vi "EditorDaemon editScript.vi"(8 "error in (no error)":errorcluster) -> (0 "error out":errorcluster)   [LabVIEW 2018]
uses:
  PC/winForms/winForms editorType.ctl
  ctl/editScriptState.ctl
  C:/ATI_MS_InstrumentControl/dll/ScintillaNET.dll
  dll/ScintillaNET.dll
  PC/PublicSubVI/Class/QMH/QMH.lvclass
  System.Windows.Forms
panel:
  in  "saveAsBtn":bool
  in  "openBtn":bool
  in  "searchStr":string caption="Search :"
  in  "script":refnum<k24>(container)
  in  "msgListbox":i32(listbox)
  in  "stop":bool
  in  "cancelBtn":bool
  in  "submitBtn":bool
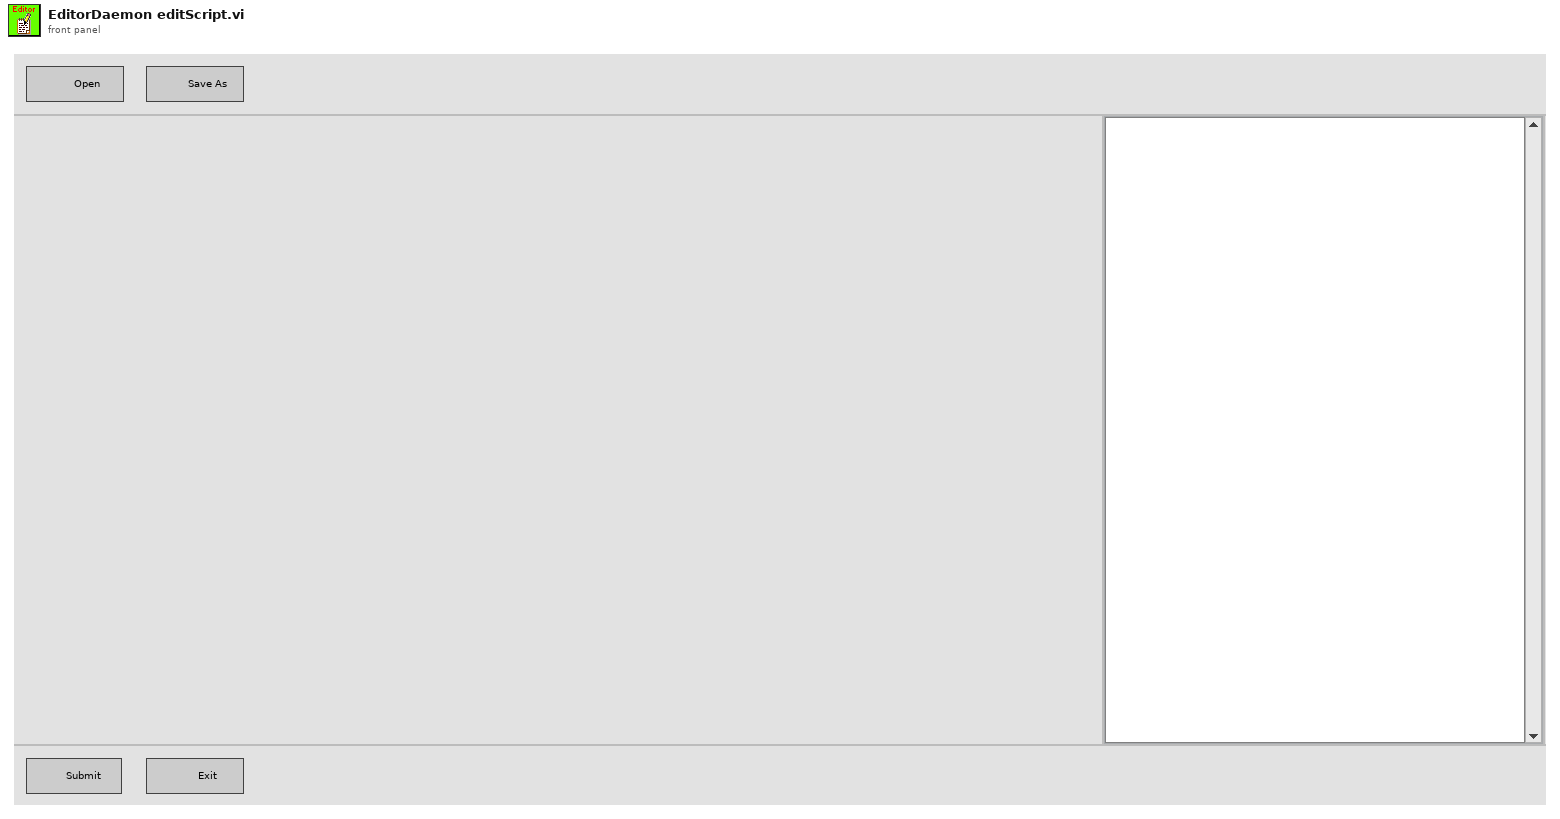
[diagram p1: front panel]
types:
  T1 = typedef "editScriptState.ctl" = enum16{"init", "loadScript", "newScript", "runScript", "close"}
  T2 = typedef "winForms editorType.ctl" = enum16{"Recipe", "SigProc", "Editor"}
  T3 = typedef "eventvkey.ctl" = enum16{"ASCII", "Enter", "Return", "Shift", "Ctrl", "Alt", "Cmd", "Opt", "Caps", "NumLock", "Clear", "Break", "Up", "Down", "Left", "Right", "Insert", "Delete", "Home", "End", "PageUp", "PageDown", "Escape", "Help", "Pause", "ScrollLock", "F1", "F2", "F3", "F4", "F5", "F6", "F7", "F8", "F9", "F10", "F11", "F12", "F13", "F14", "F15", "F16", "F17", "F18", "F19", "F20", "F21", "F22", "F23", "F24", "Play", "VolumeUp", "VolumeDown", "Mute", "Two Byte Char"}
  T4 = enum16{"open", "replace", "create", "open or create", "replace or create", "replace or create with confirmation"}
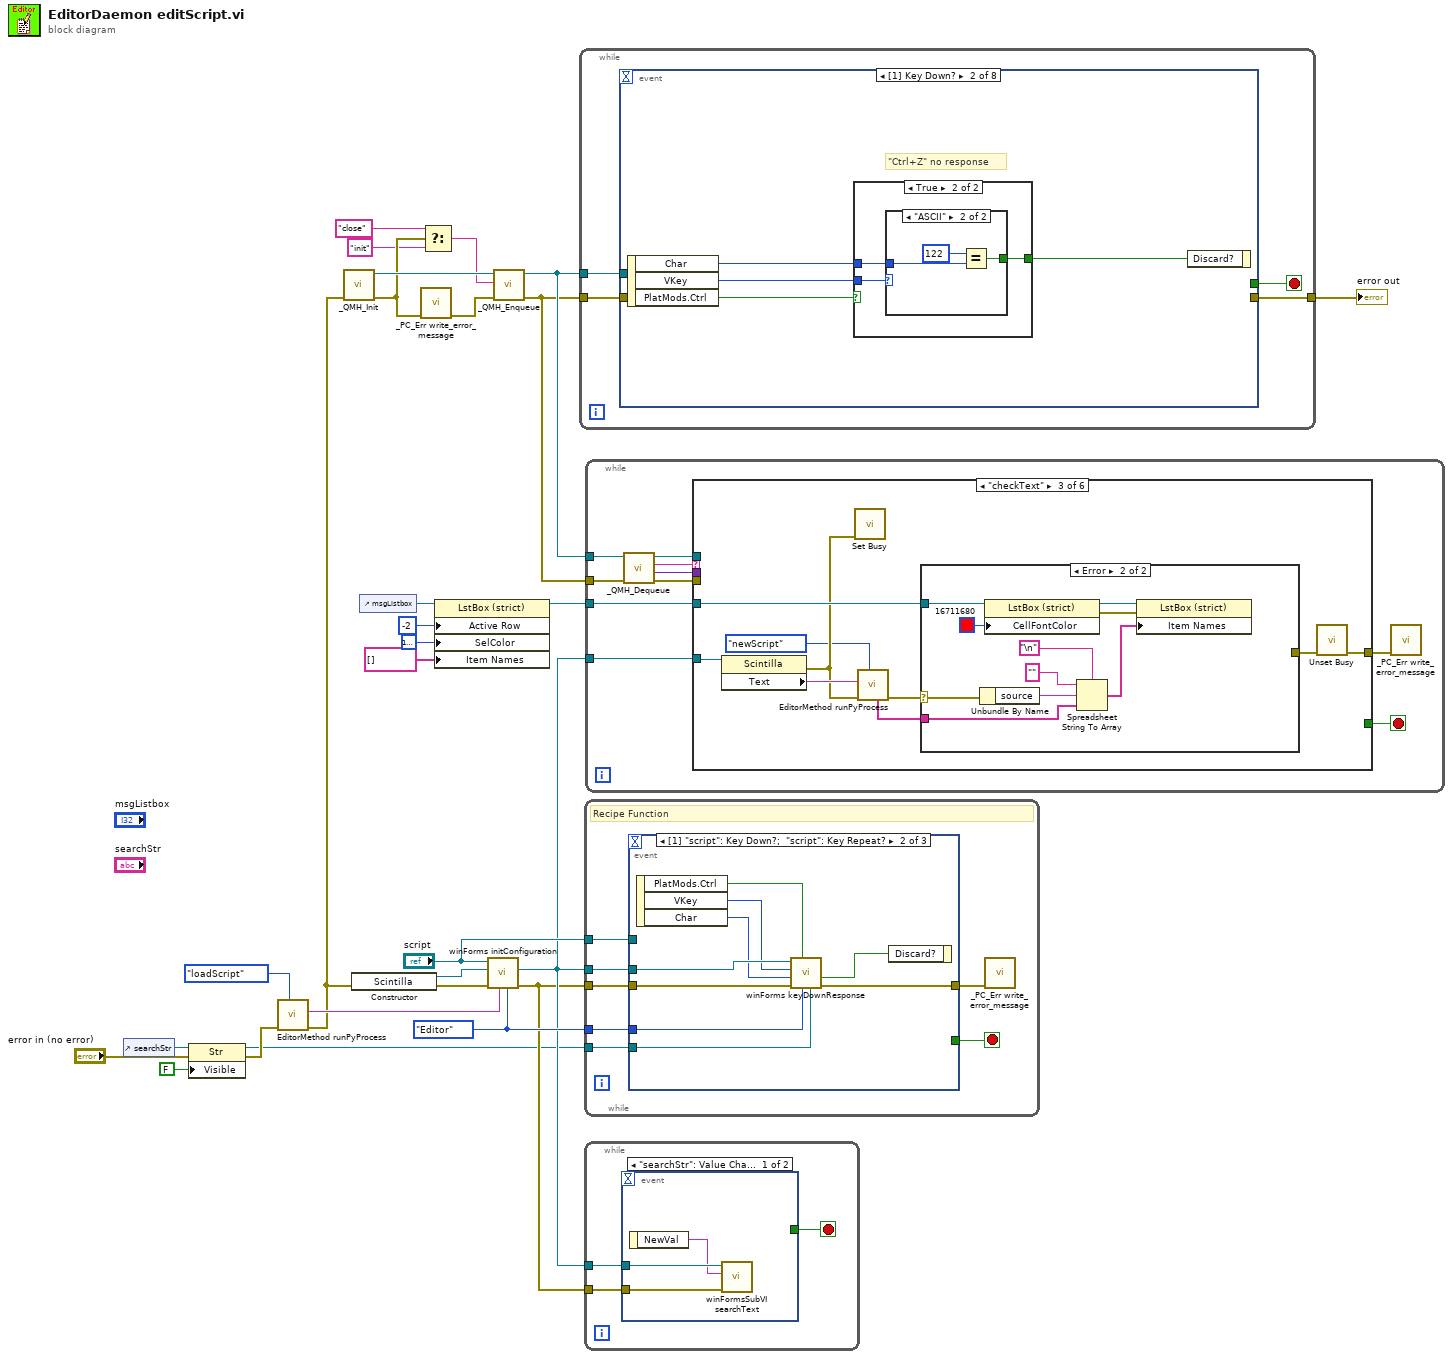
[diagram p0: block diagram]
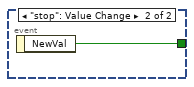
[diagram p2: hidden frame]
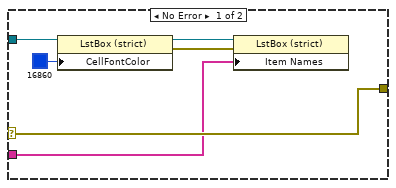
[diagram p5: hidden frame]
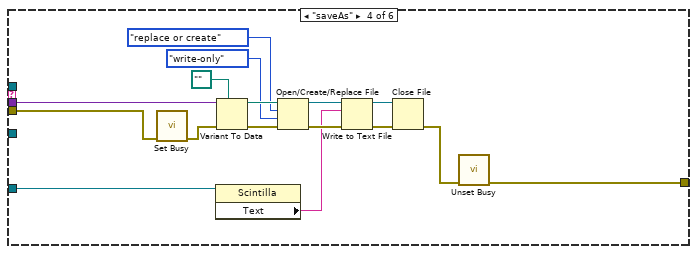
[diagram p6: hidden frame]
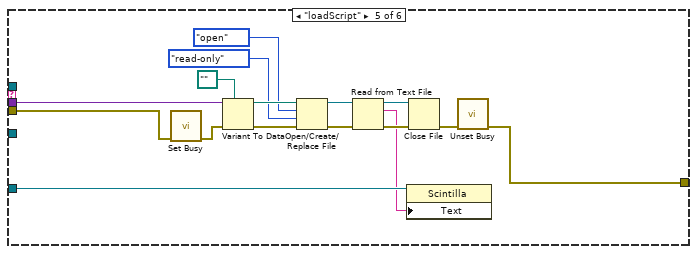
[diagram p7: hidden frame]
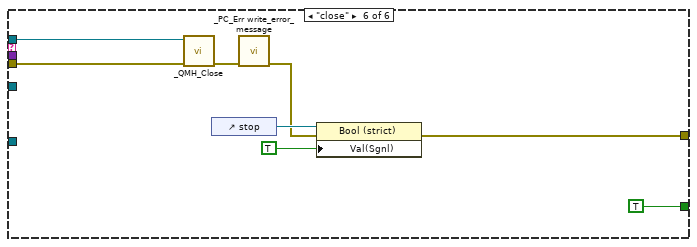
[diagram p8: hidden frame]
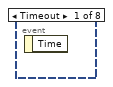
[diagram p9: hidden frame]
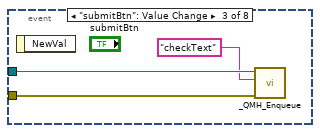
[diagram p12: hidden frame]
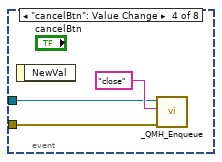
[diagram p13: hidden frame]
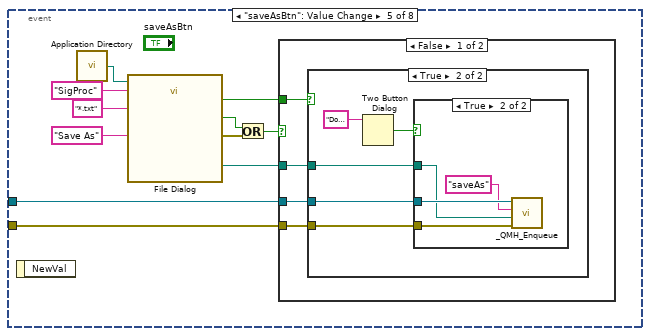
[diagram p14: hidden frame]
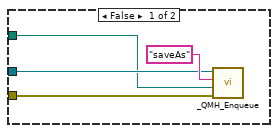
[diagram p15: hidden frame]
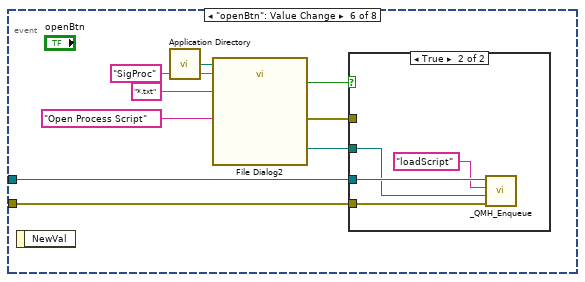
[diagram p18: hidden frame]
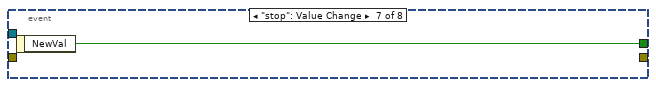
[diagram p20: hidden frame]
diagram:
  w19 = winForms_editorType."Editor" ("editorType")
  n1 = control-ref of="searchStr"() -> (w9:refnum<vi>)
  n2 = property class="Str"(reference=w9, error in="error in (no error)", "Visible"=FALSE) -> (reference out=w8:refnum<vi>, error out=w10:errorcluster)
  n3 = call "EditorMethod runPyProcess.vi"("func"=editScriptState."loadScript", "error in (no error)"=w10) -> ("error out"=w7:errorcluster, "pyCode"=w16:string)  [unwired: 6 in, 2 out]
  n4 = call "_QMH_Init.vi"("error in (no error)"=w7) -> ("error out"=w24:errorcluster, "QMH out"=w25:refnum<class "QMH.lvclass">)  [unwired: 9 in]
  n5 = constructor class="Scintilla"(error in=w7) -> (reference out=w28:refnum<k24>, error out=w27:errorcluster)  [unwired: 2 in, 1 out]
  n6 = control-ref of="msgListbox"() -> (w5:refnum<vi>)
  n7 = call "_PC_Err write_error_message.vi"("error in"=w24) -> ("error out"=w23:errorcluster)  [unwired: 10 in]
  n8 = Select(t="close", s=w24, f="init") -> (s? t:f=w22:string)
  n9 = property class="LstBox (strict)"(reference=w5, "Active Row"=-2 ("Active Row:Active Row Number"), "SelColor"=u32 16777226, "Item Names"=string[] []) -> (reference out=w4:refnum<vi>)  [unwired: 1 in, 1 out]
  n10 = call "winForms initConfiguration.vi"("editorType"=w19, "initText"=w16, "error in (no error)"=w27, "scintillaRefNum in"=w28, "panelRefNum"="script") -> ("error out"=w13:errorcluster, "scintillaRefNum out"=w14:refnum<k24>)  [unwired: 5 in]
  n11 = call "_QMH_Enqueue.vi"("error in (no error)"=w23, "Msg"=w22, "QMH in"=w25) -> ("error out"=w20:errorcluster, "QMH out"=w21:refnum<class "QMH.lvclass">)  [unwired: 7 in]
  n12 = while {
    tunnel: w21 -> [w31]
    tunnel: w20 -> [w30]
    tunnel: [w29] -> w15
    stop <- w32 stop-if-true
    n13 = event shown="[1] Key Down?" {
      selector: _ -> [_ _ _ _ _ _ _ _]
      dyn-events: _ -> [_ _ _ _ _ _ _ _]
      timeout: _ -> [_ _ _ _ _ _ _ _]
      tunnel: [_ _ _ _ _ _ w90 _] -> w32
      tunnel: w31 -> [_ _ w45 w47 w50 w78 _ w94]
      tunnel: w30 -> [_ _ w44 w46 w49 w77 _ w93]
      tunnel: [_ _ _ _ _ _ _ w91] -> w29
      event Timeout {
        n14 = event-data() -> ()  [unwired: 1 in, 1 out]
      }
      event Key Down? {
        # "\"Ctrl+Z\" no response"
        n15 = event-data() -> ("Char"=w34:i16, "VKey"=w35:T3, "PlatMods.Ctrl"=w36:bool)  [unwired: 1 in]
        n16 = case shown="True" w36 {
          tunnel: w35 -> [_ w39]
          tunnel: w34 -> [_ w38]
          tunnel: [_ w37] -> w33
          frame False {
          }
          frame True {
            n17 = case shown="\"ASCII\"" w39 {
              tunnel: w38 -> [_ w42]
              tunnel: [_ w40] -> w37
              frame "Escape", Default {
              }
              frame "ASCII" {
                n18 = Equal?(x=i16 122, y=w42) -> (x = y?=w40:bool)
              }
            }
          }
        }
        n19 = event-data("Discard?"=w33) -> ()  [unwired: 1 in, 1 out]
      }
      event "submitBtn": Value Change {
        n20 = event-data() -> ()  [unwired: 1 in, 1 out]
        n21 = call "_QMH_Enqueue.vi"("error in (no error)"=w44, "Msg"="checkText", "QMH in"=w45) -> ()  [unwired: 7 in, 2 out]
      }
      event "cancelBtn": Value Change {
        n22 = event-data() -> ()  [unwired: 1 in, 1 out]
        n23 = call "_QMH_Enqueue.vi"("error in (no error)"=w46, "Msg"="close", "QMH in"=w47) -> ()  [unwired: 7 in, 2 out]
      }
      event "saveAsBtn": Value Change {
        n24 = event-data() -> ()  [unwired: 1 in, 1 out]
        n25 = call <vilib>:"Application Directory.vi"() -> ("Application Directory"=w59:path)
        n26 = call "File Dialog"("start path"=w59, "prompt"="Save As", "default name"="SigProc" ("pattern label"), "pattern (all files)"="*.txt") -> ("selected path"=w54:path, "exists"=w55:bool, "cancelled"=w53:bool, "error out"=w52:errorcluster)  [unwired: 8 in]
        n27 = Or(x=w53, y=w52) -> (x .or. y?=w51:bool)
        n28 = case shown="False" w51 {
          tunnel: w55 -> [w63 _]
          tunnel: w54 -> [w62 _]
          tunnel: w50 -> [w61 _]
          tunnel: w49 -> [w60 _]
          frame False {
            n29 = case shown="True" w63 {
              tunnel: w62 -> [w64 w68]
              tunnel: w61 -> [w66 w70]
              tunnel: w60 -> [w65 w69]
              frame False {
                n30 = call "_QMH_Enqueue.vi"("error in (no error)"=w65, "Data"=w64, "Msg"="saveAs", "QMH in"=w66) -> ()  [unwired: 6 in, 2 out]
              }
              frame True {
                n31 = Two Button Dialog(message="Do you want to overwrite this file?") -> (T button?=w71:bool)  [unwired: 2 in]
                n32 = case shown="True" w71 {
                  tunnel: w70 -> [_ w76]
                  tunnel: w69 -> [_ w73]
                  tunnel: w68 -> [_ w75]
                  frame False {
                  }
                  frame True {
                    n33 = call "_QMH_Enqueue.vi"("error in (no error)"=w73, "Data"=w75, "Msg"="saveAs", "QMH in"=w76) -> ()  [unwired: 6 in, 2 out]
                  }
                }
              }
            }
          }
          frame True {
          }
        }
      }
      event "openBtn": Value Change {
        n34 = event-data() -> ()  [unwired: 1 in, 1 out]
        n35 = call <vilib>:"Application Directory.vi"() -> ("Application Directory"=w85:path)
        n36 = call "File Dialog2"("start path"=w85, "prompt"="Open Process Script", "default name"="SigProc" ("pattern label"), "pattern (all files)"="*.txt") -> ("selected path"=w79:path, "exists"=w81:bool, "error out"=w80:errorcluster)  [unwired: 8 in, 1 out]
        n37 = case shown="True" w81 {
          tunnel: w80 -> [_ _]
          tunnel: w79 -> [_ w86]
          tunnel: w78 -> [_ w89]
          tunnel: w77 -> [_ w88]
          frame False {
          }
          frame True {
            n38 = call "_QMH_Enqueue.vi"("error in (no error)"=w88, "Data"=w86, "Msg"="loadScript", "QMH in"=w89) -> ()  [unwired: 6 in, 2 out]
          }
        }
      }
      event "stop": Value Change {
        n39 = event-data() -> ("NewVal"=w90:bool)  [unwired: 1 in]
      }
      event Panel Close {
        n40 = event-data() -> ()  [unwired: 1 in, 1 out]
        n41 = call "_QMH_Enqueue.vi"("error in (no error)"=w93, "Msg"="close", "QMH in"=w94) -> ("error out"=w91:errorcluster)  [unwired: 7 in, 1 out]
      }
    }
  }
  "error out" <- w15
  n42 = while {
    tunnel: w14 -> [w100]
    tunnel: w13 -> [w99]
    tunnel: "script" -> [w98]
    tunnel: w19 -> [w97]
    tunnel: w8 -> [w95]
    stop <- w101 stop-if-true
    # "Recipe Function"
    n43 = event shown="[1] \"script\": Key Down?;  \"script\": Key Repeat?" {
      selector: _ -> [_ _ _]
      dyn-events: _ -> [_ _ _]
      timeout: _ -> [_ _ _]
      tunnel: [_ _ w118] -> w101
      tunnel: w100 -> [_ w110 w114]
      tunnel: w99 -> [_ w109 w113]
      tunnel: w98 -> [_ _ w116]
      tunnel: w97 -> [_ w107 _]
      tunnel: [_ w106 w115] -> w96
      tunnel: w95 -> [_ w102 _]
      event Timeout {
        n44 = event-data() -> ()  [unwired: 1 in, 1 out]
      }
      event "script": Key Down?; "script": event type 3.0.x8000000b {
        n45 = event-data() -> ("PlatMods.Ctrl"=w105:bool, "VKey"=w104:T3, "Char"=w108:i16)  [unwired: 1 in]
        n46 = call "winForms keyDownResponse.vi"("searchString"=w102, "editorType"=w107, "Ctrl"=w105, "error in (no error)"=w109, "Char"=w108, "VKey"=w104, "scintillaRefNum"=w110) -> ("error out"=w106:errorcluster, "Discard?"=w103:bool)  [unwired: 3 in]
        n47 = event-data("Discard?"=w103) -> ()  [unwired: 1 in, 1 out]
      }
      event "stop": Value Change {
        n48 = event-data() -> ("NewVal"=w118:bool)  [unwired: 1 in]
        n49 = invoke class="Scintilla" method="ClearAll"(reference=w114, error in=w113) -> (reference out=w111:refnum<k24>, error out=w112:errorcluster)  [unwired: 1 in, 1 out]
        n50 = Close Reference(reference=w111, error in (no error)=w112) -> (error out=w117:errorcluster)
        n51 = Close Reference(reference=w116, error in (no error)=w117) -> (error out=w115:errorcluster)
      }
    }
    n52 = call "_PC_Err write_error_message.vi"("error in"=w96) -> ()  [unwired: 10 in, 1 out]
  }
  n53 = while {
    tunnel: w14 -> [w121]
    tunnel: w13 -> [w120]
    stop <- w119 stop-if-true
    n54 = event shown="[0] \"searchStr\": Value Change" {
      selector: _ -> [_ _]
      dyn-events: _ -> [_ _]
      timeout: _ -> [_ _]
      tunnel: w121 -> [w124 _]
      tunnel: w120 -> [w123 _]
      tunnel: [_ w125] -> w119
      event "searchStr": Value Change {
        n55 = event-data() -> ("NewVal"=w122:string)  [unwired: 1 in]
        n56 = call "winFormsSubVI searchText.vi"("error in (no error)"=w123, "searchString"=w122, "scintillaRefNum in"=w124) -> ()  [unwired: 7 in, 2 out]
      }
      event "stop": Value Change {
        n57 = event-data() -> ("NewVal"=w125:bool)  [unwired: 1 in]
      }
    }
  }
  n58 = while {
    tunnel: w21 -> [w135]
    tunnel: w20 -> [w134]
    tunnel: w14 -> [w129]
    tunnel: w4 -> [w126]
    stop <- w127 stop-if-true
    n59 = call "_QMH_Dequeue.vi"("error in (no error)"=w134, "QMH in"=w135) -> ("error out"=w131:errorcluster, "Data"=w132:variant, "Msg"=w133:string, "QMH out"=w130:refnum<class "QMH.lvclass">)  [unwired: 4 in, 2 out]
    n60 = case shown="\"checkText\"" w133 {
      tunnel: w132 -> [_ _ _ w178 w194 _]
      tunnel: w131 -> [w136 w137 _ w170 w186 w201]
      tunnel: w130 -> [_ _ _ _ _ w202]
      tunnel: w129 -> [_ _ w146 w166 w182 _]
      tunnel: [w136 w137 w139 w167 w183 w196] -> w128
      tunnel: [_ _ _ _ _ TRUE] -> w127
      tunnel: w126 -> [_ _ w142 _ _ _]
      frame Default {
      }
      frame "init" {
      }
      frame "checkText" {
        n61 = property class="Scintilla"(reference=w146) -> (error out=w141:errorcluster, "Text"=w145:string)  [unwired: 1 in, 1 out]
        n62 = call <vilib>:"Set Busy.vi"("error in (no error)"=w141) -> ()  [unwired: 9 in, 2 out]
        n63 = call "EditorMethod runPyProcess.vi"("func"=editScriptState."newScript", "error in (no error)"=w141, "newScriptCode"=w145) -> ("error out"=w144:errorcluster, "showMsg"=w143:string[])  [unwired: 5 in, 2 out]
        n64 = case shown="Error" w144 {
          selector: w144 -> [w152 w158]
          tunnel: [w152 _] -> w140
          tunnel: w143 -> [w147 w153]
          tunnel: w142 -> [w148 w162]
          frame No Error {
            n65 = property class="LstBox (strict)"(reference=w148, "CellFontColor"=u32 16860) -> (reference out=w150:refnum<vi>, error out=w149:errorcluster)  [unwired: 1 in]
            n66 = property class="LstBox (strict)"(reference=w150, error in=w149, "Item Names"=w147) -> ()  [unwired: 2 out]
          }
          frame Error {
            n67 = Unbundle By Name(w158) -> ("source"=w156:string)
            n68 = property class="LstBox (strict)"(reference=w162, "CellFontColor"=u32 16711680) -> (reference out=w160:refnum<vi>, error out=w159:errorcluster)  [unwired: 1 in]
            n69 = Spreadsheet String To Array(delimiter (Tab)="\n", format string="", spreadsheet string=w156, array type (2D Dbl)=w153) -> (array=w154:string[])
            n70 = property class="LstBox (strict)"(reference=w160, error in=w159, "Item Names"=w154) -> ()  [unwired: 2 out]
          }
        }
        n71 = call <vilib>:"Unset Busy.vi"("error in (no error)"=w140) -> ("error out"=w139:errorcluster)  [unwired: 10 in]
      }
      frame "saveAs" {
        n72 = call <vilib>:"Set Busy.vi"("error in (no error)"=w170) -> ("error out"=w169:errorcluster)  [unwired: 9 in, 1 out]
        n73 = property class="Scintilla"(reference=w166) -> ("Text"=w165:string)  [unwired: 1 in, 2 out]
        n74 = Variant To Data(error in=w169, type=path "", Variant=w178) -> (data=w176:path, error out=w175:errorcluster)
        n75 = Open/Create/Replace File(file path (use dialog)=w176, error in=w175, operation (0:open)=T4."replace or create", access (0:read/write)=enum16{"read/write", "read-only", "write-only"}."write-only") -> (refnum out=w174:refnum<file>, error out=w173:errorcluster)  [unwired: 2 in, 1 out]
        n76 = Write to Text File(file (use dialog)=w174, text=w165, error in=w173) -> (refnum out=w172:refnum<file>, error out=w171:errorcluster)  [unwired: 1 in, 1 out]
        n77 = Close File(refnum=w172, error in=w171) -> (error out=w168:errorcluster)  [unwired: 1 out]
        n78 = call <vilib>:"Unset Busy.vi"("error in (no error)"=w168) -> ("error out"=w167:errorcluster)  [unwired: 10 in]
      }
      frame "loadScript" {
        n79 = call <vilib>:"Set Busy.vi"("error in (no error)"=w186) -> ("error out"=w185:errorcluster)  [unwired: 9 in, 1 out]
        n80 = Variant To Data(error in=w185, type=path "", Variant=w194) -> (data=w192:path, error out=w191:errorcluster)
        n81 = Open/Create/Replace File(file path (use dialog)=w192, error in=w191, operation (0:open)=T4."open", access (0:read/write)=enum16{"read/write", "read-only", "write-only"}."read-only") -> (refnum out=w190:refnum<file>, error out=w189:errorcluster)  [unwired: 2 in, 1 out]
        n82 = Read from Text File(file (use dialog)=w190, error in=w189) -> (refnum out=w188:refnum<file>, text=w181:string, error out=w187:errorcluster)  [unwired: 2 in, 1 out]
        n83 = property class="Scintilla"(reference=w182, "Text"=w181) -> ()  [unwired: 1 in, 2 out]
        n84 = Close File(refnum=w188, error in=w187) -> (error out=w184:errorcluster)  [unwired: 1 out]
        n85 = call <vilib>:"Unset Busy.vi"("error in (no error)"=w184) -> ("error out"=w183:errorcluster)  [unwired: 10 in]
      }
      frame "close" {
        n86 = call "_QMH_Close.vi"("error in (no error)"=w201, "QMH in"=w202) -> ("error out"=w198:errorcluster)  [unwired: 9 in]
        n87 = control-ref of="stop"() -> (w199:refnum<vi>)
        n88 = call "_PC_Err write_error_message.vi"("error in"=w198) -> ("error out"=w197:errorcluster)  [unwired: 10 in]
        n89 = property class="Bool (strict)"(reference=w199, error in=w197, "Val(Sgnl)"=TRUE ("Value (Signaling)")) -> (error out=w196:errorcluster)  [unwired: 1 out]
      }
    }
    n90 = call "_PC_Err write_error_message.vi"("error in"=w128) -> ()  [unwired: 10 in, 1 out]
  }
